vi "AutoDrive.vi"(6 "Reset":bool=TRUE, 7 "Distance before ultrasonic PID":dbl, 8 "error in (no error)":errorcluster, 9 "mode(T:ultrasonic,F:encoders)":bool, 10 "target":dbl, 11 "RobotDriveDevRef":T1={"DevStatus"={"status"=FALSE, "code"=0, "source"=""}, "Motors[]"=[], "Square Inputs"=FALSE, "Max Output"=1.0}) -> (0 "error out":errorcluster, 3 "RobotDriveDevRef":T1={"DevStatus"={"status"=FALSE, "code"=0, "source"=""}, "Motors[]"=[], "Square Inputs"=FALSE, "Max Output"=1.0})   [LabVIEW 2014]
uses:
  <vilib>/Rock Robotics/WPI/RobotDrive/WPI_RobotDriveDevRef.ctl
  <vilib>/Rock Robotics/WPI/MotorControl/WPI_MotorControlDeviceRef.ctl
  <vilib>/Rock Robotics/SystemInterfaces/Typedef/FPGA_TypedefDigitalModule.ctl
  <vilib>/Rock Robotics/SystemInterfaces/DIO/FPGA_DIOPWMChannel.ctl
  <vilib>/Rock Robotics/WPI/PWM/WPI_PWMDeadband.ctl
  <vilib>/Rock Robotics/WPI/CAN/Jaguar/SubVIs/WPI_CANJaguar_ControlMode.ctl
  <vilib>/Rock Robotics/WPI/PWM/WPI_PWMTransform_ConPane.ctl
  <vilib>/Rock Robotics/WPI/Ultrasonic/WPI_SonarMB1010AnalogRefNum Registry Get.vi
  <vilib>/addons/control/pid/pid.llb/PID Control Input Filter (DBL).vi
  <vilib>/addons/control/pid/pid.llb/PID (DBL).vi
  <vilib>/Rock Robotics/WPI/RobotDrive/WPI_RobotDriveArcadeDrive_Standard(NoSaturation).vi
  <vilib>/addons/control/pid/NI_PID_pid.lvlib
panel:
  out "output":dbl format="%.2f"
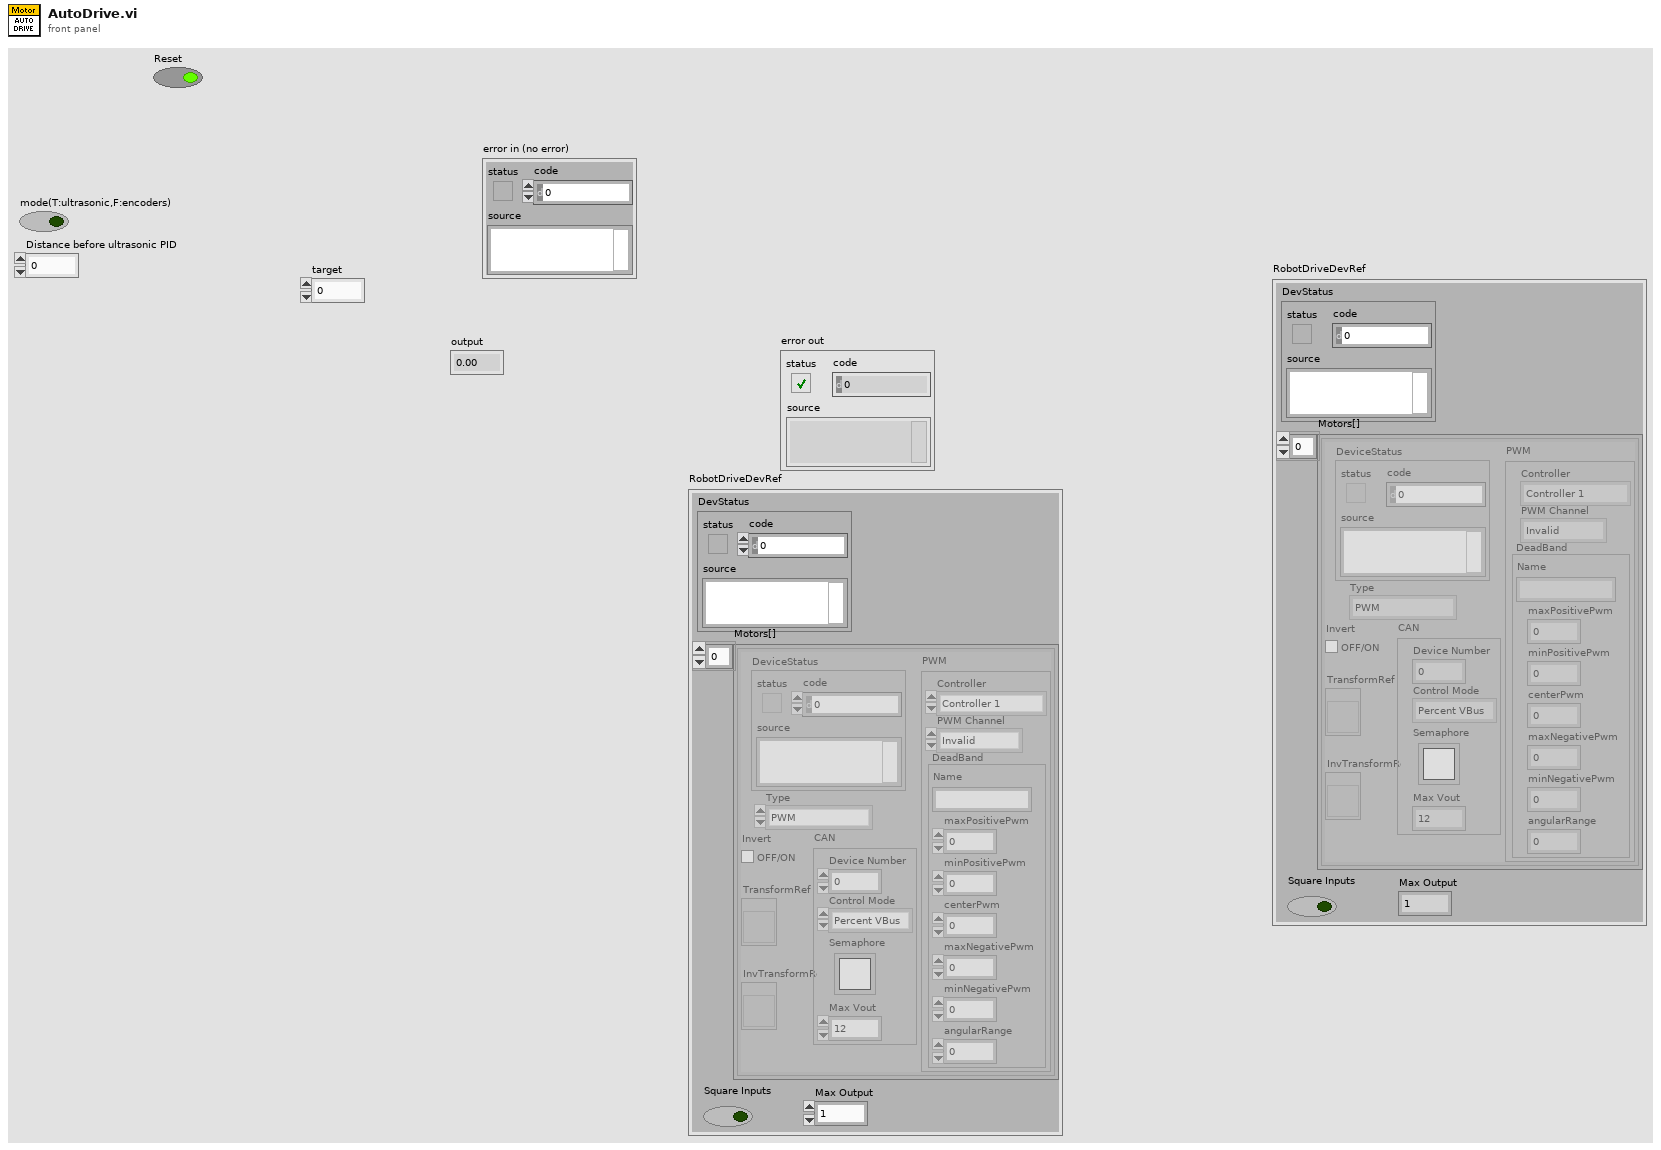
[diagram p1: front panel]
types:
  T1 = typedef "WPI_RobotDriveDevRef.ctl" = cluster{"DevStatus":errorcluster, "Motors[]":T2[], "Square Inputs":bool, "Max Output":dbl}
  T2 = typedef "WPI_MotorControlDeviceRef.ctl" = cluster{"DeviceStatus":errorcluster, "Type":enum16{"PWM", "CAN"}, "PWM":cluster{"Controller":T3, "PWM Channel":T4, "DeadBand":T5}, "CAN":cluster{"Device Number":u8, "Control Mode":T6, "Semaphore":T7, "Max Vout":dbl}, "Invert":bool, "TransformRef":T8, "InvTransformRef":T8}
  T3 = typedef "FPGA_TypedefDigitalModule.ctl" = enum16{"Controller 1"}
  T4 = typedef "FPGA_DIOPWMChannel.ctl" = enum8{"PWM 0", "PWM 1", "PWM 2", "PWM 3", "PWM 4", "PWM 5", "PWM 6", "PWM 7", "PWM 8", "PWM 9", "PWM MXP 0", "PWM MXP 1", "PWM MXP 2", "PWM MXP 3", "PWM MXP 4", "PWM MXP 5", "PWM MXP 6", "PWM MXP 7", "PWM MXP 8", "PWM MXP 9", "Invalid"}
  T5 = typedef "WPI_PWMDeadband.ctl" = cluster{"Name":string, "maxPositivePwm":i32, "minPositivePwm":i32, "centerPwm":i32, "maxNegativePwm":i32, "minNegativePwm":i32, "angularRange":u16}
  T6 = typedef "WPI_CANJaguar_ControlMode.ctl" = enum8{"Percent VBus", "Current", "Speed", "Position", "Voltage"}
  T7 = typedef "Semaphore RefNum" = refnum<k1>
  T8 = typedef "WPI_PWMTransform_ConPane.ctl" = refnum<vi>
  T9 = typedef "WPI_GyroDevRef.ctl" = cluster{"DevStatus":errorcluster, "Analog Module":T10, "Analog Channel":T11, "Offset":dbl, "Gain (VoltsPerDegree/Second)":dbl}
  T10 = typedef "FPGA_TypedefAnalogModule.ctl" = enum16{"Controller 1"}
  T11 = typedef "FPGA_AIChannel.ctl" = enum8{"AI 0", "AI 1", "AI 2", "AI 3", "AI MXP 0", "AI MXP 1", "AI MXP 2", "AI MXP 3", "Invalid"}
  T12 = typedef "WPI_SonarMB1010AnalogDeviceRef.ctl" = cluster{"AIDeviceRef":T13, "Scaling factor (V/in)":dbl, "Average Bits":u8}
  T13 = typedef "WPI_AnalogChannelDevRef.ctl" = cluster{"DevStatus":errorcluster, "Controller":T10, "Analog Channel":T11}
  T14 = typedef "WPI_EncoderDevRef.ctl" = cluster{"DevStatus":errorcluster, "EncoderIndex":T15, "CounterIndex":T16, "DistancePerCount":dbl, "Decoding Type":T17}
  T15 = typedef "FPGA_EncoderIdx.ctl" = enum8{"Enc 0", "Enc 1", "Enc 2", "Enc 3", "Invalid"}
  T16 = typedef "FPGA_CounterCtrSystemIndex.ctl" = enum8{"Ctr 0", "Ctr 1", "Ctr 2", "Ctr 3", "Ctr 4", "Ctr 5", "Ctr 6", "Ctr 7", "Invalid"}
  T17 = typedef "WPI_EncoderType.ctl" = enum16{"1x", "2x", "4x"}
  T18 = cluster{"proportional gain (Kc)":dbl, "integral time (Ti, min)":dbl, "derivative time (Td, min)":dbl}
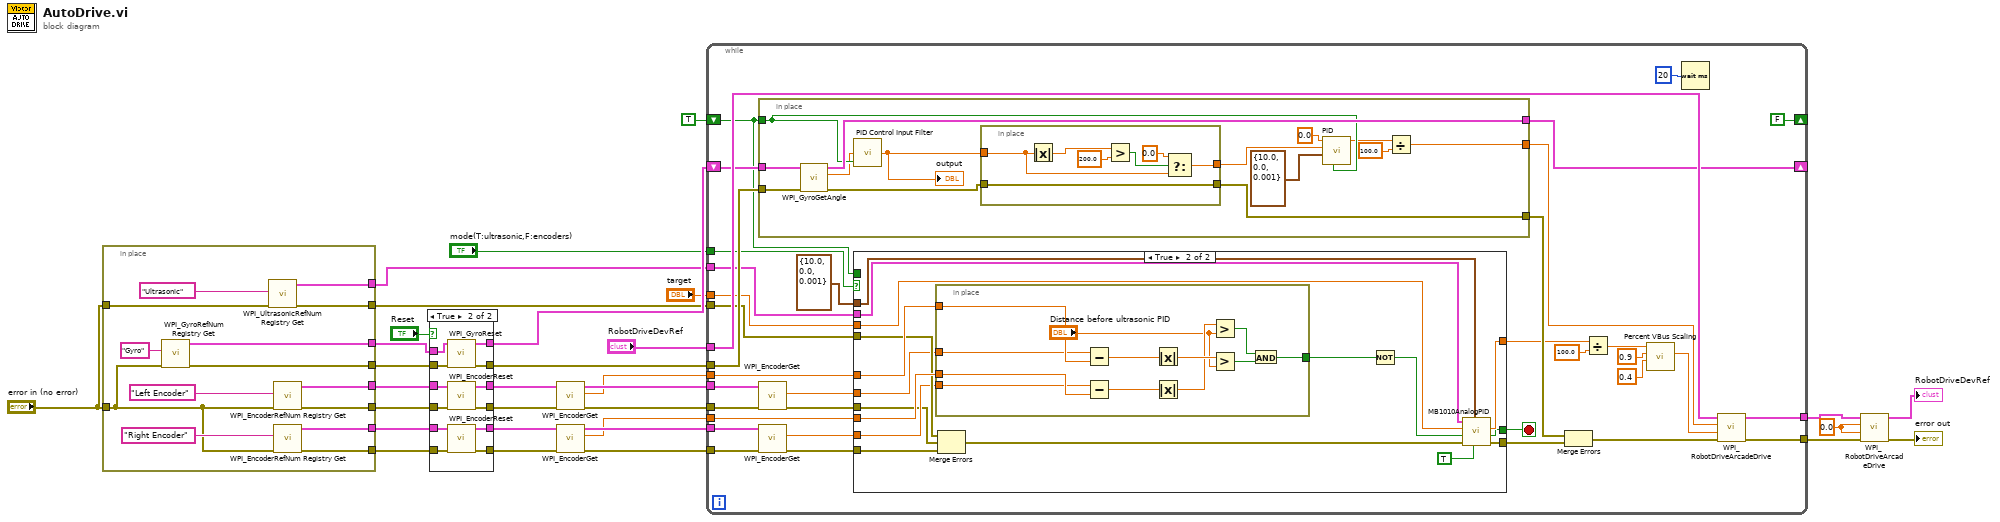
[diagram p0: block diagram]
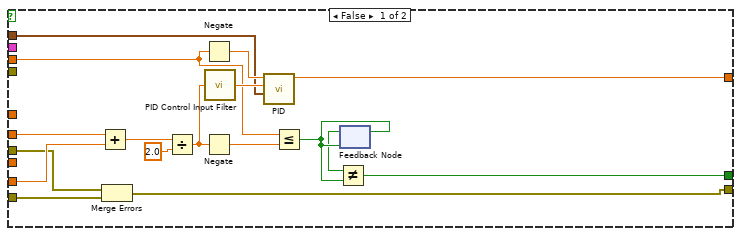
[diagram p2: hidden frame]
diagram:
  w26 = 0.0 ("X axis value")
  n1 = in-place {
    in-place-border: "error in (no error)" -> [w38]
    in-place-border: [w45] -> w23
    in-place-border: [w44] -> w22
    in-place-border: [w37] -> w18
    in-place-border: [w39] -> w15
    in-place-border: [w36] -> w19
    in-place-border: [w40] -> w16
    in-place-border: "error in (no error)" -> [w34]
    in-place-border: [w33] -> w2
    in-place-border: [w32] -> w1
    n2 = call <vilib>:"WPI_GyroRefNum Registry Get.vi"("error in (no error)"=w38, "refnum name"="Gyro") -> ("error out"=w45:errorcluster, "GyroDevRef"=w44:T9)  [unwired: 8 in]
    n3 = call-poly <vilib>:"WPI_UltrasonicRefNum Registry Get.vi"("error in (no error)"=w34, "refnum name"="Ultrasonic") -> ("error out"=w33:errorcluster, "SonarMB1010AnalogDevRef"=w32:T12)  [unwired: 8 in]
    n4 = call <vilib>:"WPI_EncoderRefNum Registry Get.vi"("error in (no error)"=w38, "refnum name"="Left Encoder") -> ("error out"=w39:errorcluster, "EncoderDevRef"=w36:T14)  [unwired: 8 in]
    n5 = call <vilib>:"WPI_EncoderRefNum Registry Get.vi"("error in (no error)"=w38, "refnum name"="Right Encoder") -> ("error out"=w40:errorcluster, "EncoderDevRef"=w37:T14)  [unwired: 8 in]
  }
  n6 = case shown="True" "Reset" {
    tunnel: w22 -> [w51 w63]
    tunnel: w23 -> [w50 w62]
    tunnel: [w50 w61] -> w24
    tunnel: [w51 w60] -> w25
    tunnel: w16 -> [w49 w52]
    tunnel: w19 -> [w47 w59]
    tunnel: w18 -> [w48 w58]
    tunnel: [w49 w57] -> w10
    tunnel: [w48 w55] -> w11
    tunnel: [w47 w56] -> w12
    tunnel: [w46 w54] -> w13
    tunnel: w15 -> [w46 w53]
    frame False {
    }
    frame True {
      n7 = call <vilib>:"WPI_GyroReset.vi"("error in (no error)"=w62, "GyroDevRef"=w63) -> ("error out"=w61:errorcluster, "GyroDevRef"=w60:T9)  [unwired: 8 in]
      n8 = call <vilib>:"WPI_EncoderReset.vi"("error in (no error)"=w53, "EncoderDevRef"=w59) -> ("error out"=w54:errorcluster, "EncoderDevRef"=w56:T14)  [unwired: 8 in]
      n9 = call <vilib>:"WPI_EncoderReset.vi"("error in (no error)"=w52, "EncoderDevRef"=w58) -> ("error out"=w57:errorcluster, "EncoderDevRef"=w55:T14)  [unwired: 8 in]
    }
  }
  n10 = call <vilib>:"WPI_EncoderGet.vi"("error in (no error)"=w13, "EncoderDevRef"=w12) -> ("error out"=w7:errorcluster, "Distance"=w5:dbl, "EncoderDevRef"=w6:T14)  [unwired: 4 in, 3 out]
  n11 = call <vilib>:"WPI_EncoderGet.vi"("error in (no error)"=w10, "EncoderDevRef"=w11) -> ("error out"=w9:errorcluster, "Distance"=w4:dbl, "EncoderDevRef"=w8:T14)  [unwired: 4 in, 3 out]
  n12 = while {
    tunnel: [w98] -> w17
    tunnel: [w97] -> w27
    tunnel: "RobotDriveDevRef" -> [w96]
    tunnel: w24 -> [w94]
    tunnel: w2 -> [w86]
    shift-right: [FALSE] -> _
    shift-left: TRUE -> [w89]
    tunnel: "target" -> [w91]
    shift-right: [w90] -> _
    shift-left: w25 -> [w95]
    tunnel: w9 -> [w68]
    tunnel: w7 -> [w71]
    tunnel: w8 -> [w73]
    tunnel: w6 -> [w70]
    tunnel: w1 -> [w87]
    tunnel: "mode(T:ultrasonic,F:encoders)" -> [w82]
    tunnel: w5 -> [w75]
    tunnel: w4 -> [w74]
    stop <- w64 stop-if-true
    n13 = in-place {
      in-place-border: w95 -> [w158]
      in-place-border: w94 -> [w157]
      in-place-border: [w156] -> w90
      in-place-border: w89 -> [w155]
      in-place-border: [w147] -> w85
      in-place-border: [w145] -> w84
      n14 = call <vilib>:"WPI_GyroGetAngle.vi"("error in (no error)"=w157, "GyroDevRef"=w158) -> ("error out"=w146:errorcluster, "Angle"=w154:dbl, "GyroDevRef"=w156:T9)  [unwired: 6 in, 1 out]
      n15 = call-poly <vilib>:"PID Control Input Filter.vi"("reinitialize? (F)"=w155, "input"=w154) -> ("output"=w149:dbl)  [unwired: 3 in]
      "output" <- w149
      n16 = in-place {
        in-place-border: w149 -> [w162]
        in-place-border: [w163] -> w148
        in-place-border: w146 -> [w159]
        in-place-border: [w159] -> w145
        n17 = Absolute Value(x=w162) -> (abs(x)=w165:dbl)
        n18 = Greater?(x=w165, y=200.0) -> (0:w160:bool)
        n19 = Select(t=0.0 ("f"), s=w160, f=w162) -> (s? t:f=w163:dbl)
      }
      n20 = call-poly <vilib>:"PID.vi"("reinitialize? (F)"=w155, "PID gains"=T18 {"proportional gain (Kc)"=10.0, "integral time (Ti, min)"=0.0, "derivative time (Td, min)"=0.001} ("X PID gains"), "process variable"=w148, "setpoint"=0.0) -> ("output"=w153:dbl)  [unwired: 6 in, 1 out]
      n21 = Divide(x=w153, y=100.0) -> (x/y=w147:dbl)
    }
    n22 = call <vilib>:"WPI_EncoderGet.vi"("error in (no error)"=w71, "EncoderDevRef"=w70) -> ("error out"=w67:errorcluster, "Distance"=w69:dbl)  [unwired: 4 in, 4 out]
    n23 = call <vilib>:"WPI_EncoderGet.vi"("error in (no error)"=w68, "EncoderDevRef"=w73) -> ("error out"=w66:errorcluster, "Distance"=w72:dbl)  [unwired: 4 in, 4 out]
    n24 = case shown="True" w82 {
      tunnel: w91 -> [w109 w127]
      tunnel: w89 -> [_ _]
      tunnel: w87 -> [_ w116]
      tunnel: w86 -> [_ w129]
      tunnel: [w103 w126] -> w78
      tunnel: [w105 w117] -> w64
      tunnel: [w106 w120] -> w83
      tunnel: T18 {"proportional gain (Kc)"=10.0, "integral time (Ti, min)"=0.0, "derivative time (Td, min)"=0.001} ("PID gains") -> [w104 w130]
      tunnel: w75 -> [_ w132]
      tunnel: w74 -> [_ w131]
      tunnel: w72 -> [w102 w125]
      tunnel: w69 -> [w101 w124]
      tunnel: w67 -> [w100 w121]
      tunnel: w66 -> [w99 w122]
      frame False {
        n25 = Add(x=w101, y=w102) -> (x+y=w112:dbl)
        n26 = Merge Errors(w100, w99) -> (w106:errorcluster)
        n27 = Divide(x=w112, y=2.0) -> (x/y=w114:dbl)
        n28 = Negate(x=w109) -> (-x=w115:dbl)
        n29 = Negate(x=w114) -> (-x=w108:dbl)
        n30 = call-poly <vilib>:"PID Control Input Filter.vi"("input"=w114) -> ("output"=w111:dbl)  [unwired: 4 in]
        n31 = call-poly <vilib>:"PID.vi"("PID gains"=w104, "process variable"=w111, "setpoint"=w115) -> ("output"=w103:dbl)  [unwired: 7 in, 1 out]
        n32 = Less Or Equal?(x=w109, y=w108) -> (x <= y?=w110:bool)
        n33 = feedback #1(w110) -> (w107:bool)
        n34 = Not Equal?(x=w107, y=w110) -> (x != y?=w105:bool)
        n35 = feedback-in #1(w110) -> ()
      }
      frame True {
        n36 = in-place {
          in-place-border: [w140] -> w128
          in-place-border: w132 -> [w138]
          in-place-border: w131 -> [w136]
          in-place-border: w125 -> [w134]
          in-place-border: w124 -> [w133]
          n37 = Subtract(x=w133, y=w138) -> (x-y=w139:dbl)
          n38 = Subtract(x=w134, y=w136) -> (x-y=w137:dbl)
          n39 = Absolute Value(x=w139) -> (abs(x)=w144:dbl)
          n40 = Absolute Value(x=w137) -> (abs(x)=w143:dbl)
          n41 = Greater?(x=w143, y="Distance before ultrasonic PID") -> (0:w142:bool)
          n42 = Greater?(x=w144, y="Distance before ultrasonic PID") -> (0:w141:bool)
          n43 = And(x=w142, y=w141) -> (x .and. y?=w140:bool)
        }
        n44 = Merge Errors(w129, w121, w122) -> (w123:errorcluster)
        n45 = Not(x=w128) -> (.not. x?=w118:bool)
        n46 = call "MB1010AnalogPID.vi"("Forward"=TRUE, "PID gains"=w130, "error in (no error)"=w123, "FullSpeed"=w118, "setpoint"=w127, "SonarMB1010AnalogDevRef"=w116) -> ("error out"=w120:errorcluster, "CrossedSetpoint"=w117:bool, "output"=w126:dbl)  [unwired: 2 in, 1 out]
      }
    }
    n47 = Merge Errors(w84, w83) -> (w88:errorcluster)
    n48 = Divide(x=w78, y=100.0) -> (x/y=w80:dbl)
    n49 = call "Percent VBus Scaling.vi"("Min %VBus"=0.4, "Max %VBus"=0.9, "input (1 to -1)"=w80) -> ("output"=w65:dbl)  [unwired: 8 in]
    n50 = Wait (ms)(milliseconds to wait=u32 20) -> ()  [unwired: 1 out]
    n51 = call-poly <vilib>:"WPI_RobotDriveArcadeDrive.vi"("error in (no error)"=w88, "Y axis value"=w65, "X axis value"=w85, "RobotDriveDevRef"=w96) -> ("error out"=w98:errorcluster, "RobotDriveDevRef"=w97:T1)  [unwired: 5 in, 1 out]
  }
  n52 = call-poly <vilib>:"WPI_RobotDriveArcadeDrive.vi"("error in (no error)"=w17, "Y axis value"=w26, "X axis value"=w26, "RobotDriveDevRef"=w27) -> ("error out"=→"error out":errorcluster, "RobotDriveDevRef"=→"RobotDriveDevRef":T1)  [unwired: 5 in, 1 out]
